vi "Handle setConfiguration.vi"(8 "error in (no error)":errorcluster, 10 "setConfiguration":variant, 11 "Inst.FP in":refnum<class "Inst.FP.lvclass">) -> (0 "error out":errorcluster, 3 "Inst.FP out":refnum<class "Inst.FP.lvclass">)   [LabVIEW 2019, in "Inst.FP.lvclass"]
uses:
  Inst.FP.lvclass
  Inst.FP.lvclass/Inst.FP.ctl
  45e4b271-6884-462c-ad3a-d505ab08eb62.vi
  45e4b271-6884-462c-ad3a-d505ab08eb62.vi/af630d1c-820b-4575-90bf-b645f106faf9.vi
  45e4b271-6884-462c-ad3a-d505ab08eb62.vi/04fe8b5c-4c70-4330-9607-ed929486d21b.vi
  <vilib>/Utility/Data Type/Get Type Information.vi
  <vilib>/JDP Science/JSONtext/JSON text to Variant.vi
  <vilib>/JDP Science/JSONtext/LVClass Serializer/JSONtext LVClass Serializer.lvclass
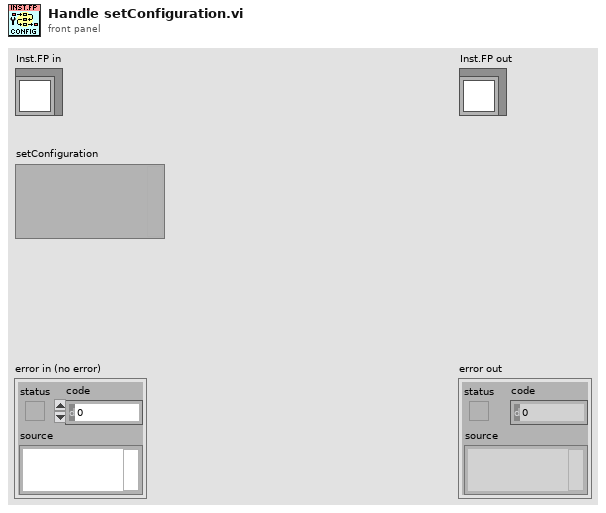
[diagram p1: front panel]
types:
  T1 = typedef "Inst.FP.lvclass/Inst.FP.Configuration--Cluster.ctl" = cluster{"FP Type":T2}
  T2 = typedef "Inst.FP.lvclass/Inst.FP.Type--Enum.ctl" = enum32{"Wet", "CF"}
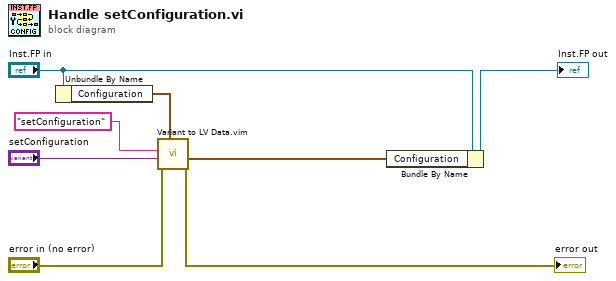
[diagram p0: block diagram]
diagram:
  n1 = Unbundle By Name("Inst.FP in") -> ("Configuration"=w7:T1)
  n2 = call "Variant to LV Data.vim"("type"=w7, "error in (no error)"="error in (no error)", "JSON Data in"="setConfiguration", "Command"="setConfiguration") -> ("error out"=→"error out":errorcluster, "Data out"=w1:T1)  [unwired: 4 in, 2 out]
  n3 = Bundle By Name(cluster="Inst.FP in", "Configuration"=w1) -> (→"Inst.FP out":refnum<class "Inst.FP.lvclass">)
